vi "Is Runtime Application.vi"(3 "error in":errorcluster) -> (7 "Runtime ?":bool, 9 "error out":errorcluster)   [LabVIEW 2021, in "Utilities.lvlib"]
uses:
  Utilities.lvlib
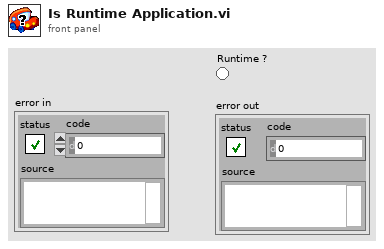
[diagram p1: front panel]
types:
  T1 = enum32{"invalid app kind", "Development System", "Run Time System", "Student Edition", "Embedded LabVIEW", "Evaluation", "Custom"}
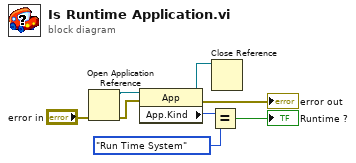
[diagram p0: block diagram]
diagram:
  n1 = Open Application Reference(8:"error in") -> (0:w6:errorcluster, 3:w4:refnum<vi>)  [unwired: 3 in]
  n2 = property class="App"(reference=w4, error in=w6) -> (reference out=w8:refnum<vi>, error out=→"error out":errorcluster, "App.Kind"=w1:T1)
  n3 = Equal?(x=w1, y=T1."Run Time System" ("Application:Kind")) -> (x = y?=→"Runtime ?":bool)
  n4 = Close Reference(reference=w8) -> ()  [unwired: 1 in, 1 out]
